vi "sub_system_status.vi"(7 "Mode":enum16{"Initial", "Update", "Clear"}(ring)=enum."Update", 8 "에러 입력(에러 없음)":errorcluster, 10 "String in":string, 11 "System Log":refnum<vi>) -> (0 "에러 출력":errorcluster)   [LabVIEW 2016]
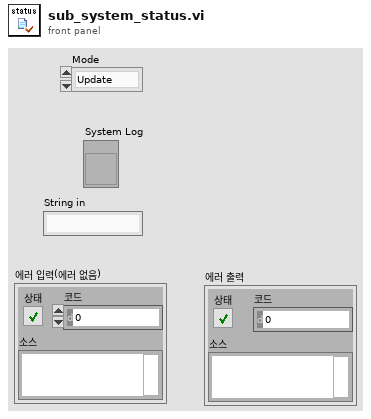
[diagram p1: front panel]
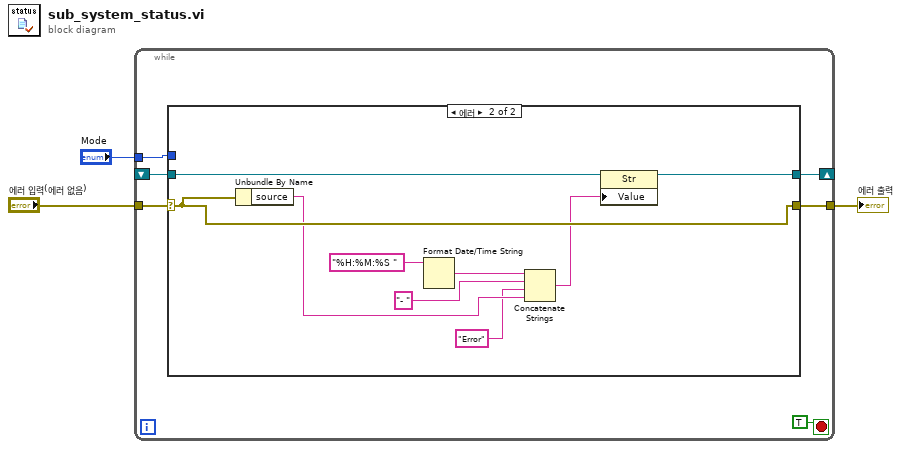
[diagram p0: block diagram]
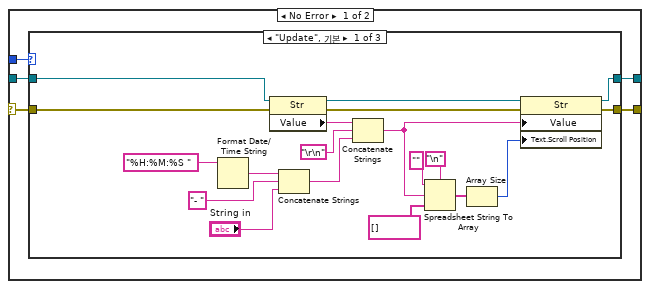
[diagram p2: hidden frame]
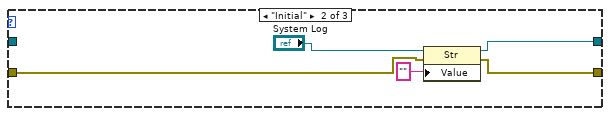
[diagram p3: hidden frame]
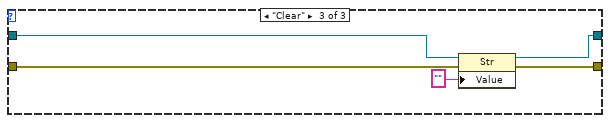
[diagram p4: hidden frame]
diagram:
  n1 = while {
    tunnel: "에러 입력(에러 없음)" -> [w4]
    tunnel: [w9] -> w2
    tunnel: "Mode" -> [w7]
    shift-right: [w6] -> _
    shift-left: _ -> [w5]
    stop <- TRUE stop-if-true
    n2 = case shown="에러" w4 {
      selector: w4 -> [w10 w50]
      tunnel: [w14 w50] -> w9
      tunnel: w7 -> [w13 _]
      tunnel: [w12 w51] -> w6
      tunnel: w5 -> [w11 w52]
      frame No Error {
        n3 = case shown="\"Update\", 기본" w13 {
          tunnel: w11 -> [w33 _ w41]
          tunnel: w10 -> [w28 w35 w43]
          tunnel: [w27 w36 w42] -> w14
          tunnel: [w26 w37 w40] -> w12
          frame "Update", Default {
            n4 = Format Date/Time String(time format string (%c)="%H:%M:%S " ("시간 포맷 문자열 (%c)")) -> (date/time string=w18:string)  [unwired: 2 in]
            n5 = property class="Str"(reference=w33, error in=w28) -> (reference out=w30:refnum<vi>, error out=w29:errorcluster, "Value"=w32:string)
            n6 = Concatenate Strings(w18, "- " ("포맷 문자열"), "String in") -> (w17:string)
            n7 = Concatenate Strings(w32, "\r\n", w17) -> (w21:string)
            n8 = Spreadsheet String To Array(delimiter (Tab)="\n", format string="" ("포맷 문자열"), spreadsheet string=w21, array type (2D Dbl)=string[] []) -> (array=w25:string[])
            n9 = Array Size(array=w25) -> (size(s)=w20:i32)
            n10 = property class="Str"(reference=w30, error in=w29, "Value"=w21, "Text.Scroll Position"=w20) -> (reference out=w26:refnum<vi>, error out=w27:errorcluster)
          }
          frame "Initial" {
            n11 = property class="Str"(reference="System Log", error in=w35, "Value"="" ("값")) -> (reference out=w37:refnum<vi>, error out=w36:errorcluster)
          }
          frame "Clear" {
            n12 = property class="Str"(reference=w41, error in=w43, "Value"="" ("값")) -> (reference out=w40:refnum<vi>, error out=w42:errorcluster)
          }
        }
      }
      frame Error {
        n13 = Unbundle By Name(w50) -> ("source"=w45:string)
        n14 = Format Date/Time String(time format string (%c)="%H:%M:%S " ("시간 포맷 문자열 (%c)")) -> (date/time string=w48:string)  [unwired: 2 in]
        n15 = Concatenate Strings(w48, "- " ("포맷 문자열"), "Error" ("문자열"), w45) -> (w46:string)
        n16 = property class="Str"(reference=w52, "Value"=w46) -> (reference out=w51:refnum<vi>)  [unwired: 1 in, 1 out]
      }
    }
  }
  "에러 출력" <- w2
